vi "Read Waveform (Single).vi"(8 "error in (no error)":errorcluster, 9 "Maximum Time (10000 ms)":u32=10000, 10 "Channel (1: Channel 1)":u16(ring)=1 items=["Channel 1"=1, "Channel 2"=2], 11 "VISA resource name":refnum<visa-resource-name>) -> (0 "error out":errorcluster, 2 "Waveform Data":waveform(dbl)(graph), 3 "VISA resource name out":refnum<visa-resource-name>)   [LabVIEW 2020, in "Template - Scope.lvlib"]
doc: "Initiates an acquisition on all channels that you enabled with the <b>Configure Channel</b> VI. The VI waits for the acquisition to complete and returns the waveform for the <b>Source Channel</b> you specified. If the oscilloscope did not complete the acquisition within the time period you specify with the <b>Timeout</b> control, the VI returns a timeout error. A common cause for a timeout error is the acquisition was not triggered. For example, the trigger level is out of range of the waveform.\n\nCall the <b>Fetch Waveform</b> VI to obtain the waveforms for each of the remaining enabled <b>Source Channels</b> without initiating another acquisition.\n\n<b>Note:</b> If your instrument does not support auto compensation for probe attenuation, you may need to adjust the scaling of the Waveform Data accordingly. This is handled automatically in the <b>Configure Channel</b> VI or can be done manually by multiplying the <b>Waveform Data</b> by the probe attenuation."
uses:
  <instrlib>/_Template - Scope/Template - Scope.lvlib
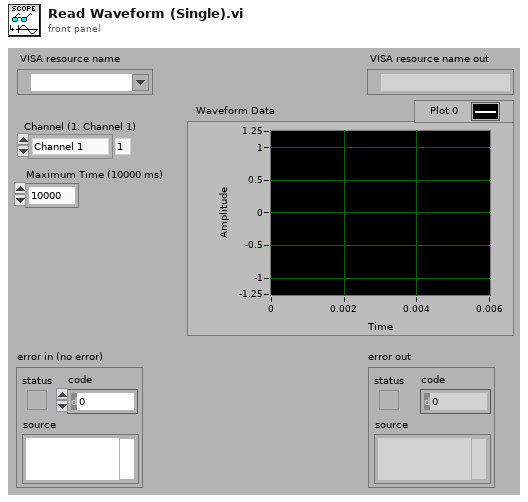
[diagram p1: front panel]
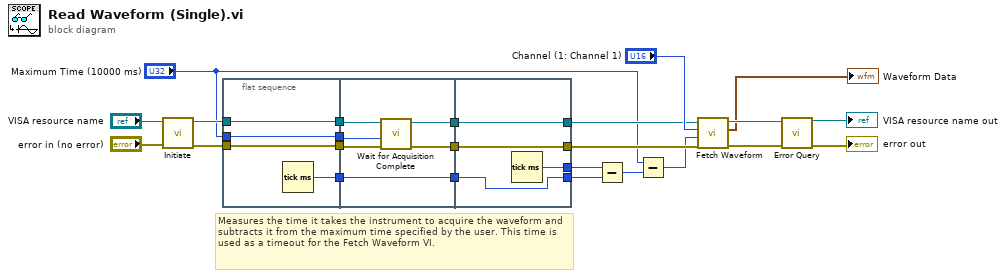
[diagram p0: block diagram]
diagram:
  # "Measures the time it takes the instrument to acquire the waveform and subtracts it from the maximum time specified by the user. This time is used as a timeout for the Fetch Waveform VI."
  n1 = call <instrlib>:"Initiate.vi"("error in (no error)"="error in (no error)", "VISA resource name"="VISA resource name") -> ("error out"=w14:errorcluster, "VISA resource name out"=w16:refnum<visa-resource-name>)  [unwired: 8 in]
  n2 = flat-sequence {
    tunnel: w16 -> [w27]
    tunnel: [w27] -> w7
    tunnel: w14 -> [w26]
    tunnel: [w26] -> w6
    tunnel: "Maximum Time (10000 ms)" -> [w25]
    tunnel: [w25] -> w5
    tunnel: [w28] -> w4
    tunnel: w7 -> [w34]
    tunnel: [w33] -> w3
    tunnel: w6 -> [w32]
    tunnel: [w31] -> w2
    tunnel: w5 -> [w30]
    tunnel: w4 -> [w29]
    tunnel: [w29] -> w1
    tunnel: [w37] -> w15
    tunnel: w3 -> [w37]
    tunnel: [w36] -> w13
    tunnel: w2 -> [w36]
    tunnel: [w35] -> w9
    tunnel: w1 -> [w35]
    tunnel: [w38] -> w8
    frame #0 {
      n3 = Tick Count (ms)() -> (millisecond timer value=w28:u32)
    }
    frame #1 {
      n4 = call <instrlib>:"Wait for Acquisition Complete.vi"("error in (no error)"=w32, "Maximum Time (10000 ms)"=w30, "VISA resource name"=w34) -> ("error out"=w31:errorcluster, "VISA resource name out"=w33:refnum<visa-resource-name>)  [unwired: 7 in]
    }
    frame #2 {
      n5 = Tick Count (ms)() -> (millisecond timer value=w38:u32)
    }
  }
  n6 = Subtract(x=w8, y=w9) -> (x-y=w12:u32)
  n7 = Subtract(x="Maximum Time (10000 ms)", y=w12) -> (x-y=w10:u32)
  n8 = call <instrlib>:"Fetch Waveform.vi"("error in (no error)"=w13, "Timeout (10000 ms)"=w10, "Channel (1: Channel 1)"="Channel (1: Channel 1)", "VISA resource name"=w15) -> ("error out"=w18:errorcluster, "Waveform Data"=→"Waveform Data":waveform(dbl), "VISA resource name out"=w19:refnum<visa-resource-name>)  [unwired: 5 in]
  n9 = call <instrlib>:"Error Query.vi"("error in (no error)"=w18, "VISA resource name"=w19) -> ("error out"=→"error out":errorcluster, "VISA resource name out"=→"VISA resource name out":refnum<visa-resource-name>)  [unwired: 6 in, 2 out]
